vi "2ndContollerStatus.vi"() -> ()   [LabVIEW 2016]
panel:
  out "shooterStatus":bool
  out "intakeStatus":bool
  out "gearStatus":bool
  out "controllerStatus":dbl
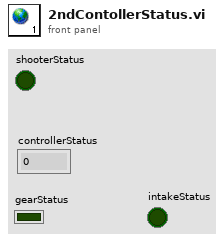
[diagram p1: front panel]
diagram:
